vi "SICMDisplayGraph.vi"(6 "Baseline":dbl, 7 "Data":i16[](array[numeric]), 8 "TriggerHeight":dbl, 9 "TimeRes":cluster{"feedbackHz":u32, "memorywWriteDec":u16}, 10 "voltageRange":dbl, 11 "ArrayToReplace":waveform(dbl)[](array[waveform])) -> (3 "Graph":waveform(dbl)[](array[waveform]))   [LabVIEW 2016]
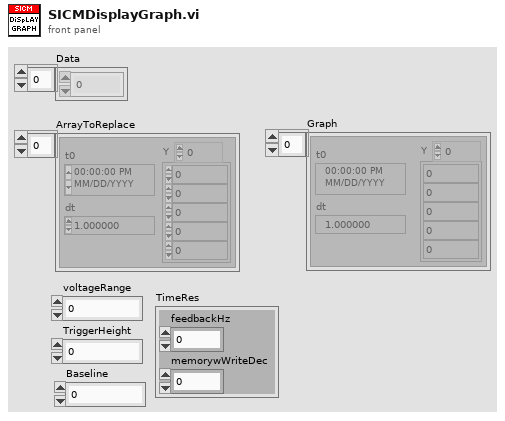
[diagram p1: front panel]
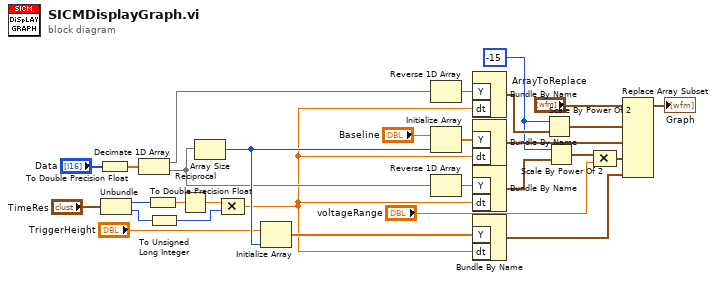
[diagram p0: block diagram]
diagram:
  w8 = i16 -15 ("n")
  n1 = To Double Precision Float(number="Data") -> (double precision float=w21:dbl[])
  n2 = Unbundle("TimeRes") -> ("feedbackHz"=w4:u32, "memorywWriteDec"=w2:u16)
  n3 = Decimate 1D Array(w21) -> (w11:dbl[], w13:dbl[])
  n4 = To Double Precision Float(number=w4) -> (double precision float=w7:dbl)
  n5 = To Unsigned Long Integer(number=w2) -> (unsigned 32bit integer=w1:u32)
  n6 = Reciprocal(x=w7) -> (1/x=w6:dbl)
  n7 = Array Size(array=w13) -> (size(s)=w15:i32)
  n8 = Compound Arithmetic op=MULTIPLY(w6, w1) -> (w3:dbl)
  n9 = Initialize Array("TriggerHeight", w15) -> (w18:dbl[])
  n10 = Reverse 1D Array(array=w11) -> (reversed array=w23:dbl[])
  n11 = Initialize Array("Baseline", w15) -> (w12:dbl[])
  n12 = Reverse 1D Array(array=w13) -> (reversed array=w24:dbl[])
  n13 = Bundle By Name("Y"=w23, "dt"=w3) -> (w19:waveform(dbl))  [unwired: 1 in]
  n14 = Bundle By Name("Y"=w12, "dt"=w3) -> (w27:waveform(dbl))  [unwired: 1 in]
  n15 = Bundle By Name("Y"=w24, "dt"=w3) -> (w20:waveform(dbl))  [unwired: 1 in]
  n16 = Bundle By Name("Y"=w18, "dt"=w3) -> (w26:waveform(dbl))  [unwired: 1 in]
  n17 = Scale By Power Of 2(n=w8, x=w19) -> (x*2^n=w28:waveform(dbl))
  n18 = Scale By Power Of 2(n=w8, x=w20) -> (x*2^n=w17:waveform(dbl))
  n19 = Compound Arithmetic op=MULTIPLY(w17, "voltageRange") -> (w25:waveform(dbl))
  n20 = Replace Array Subset(array="ArrayToReplace", new element #1=w28, new element #2=w27, new element #3=w25, new element #4=w26) -> (→"Graph":waveform(dbl)[])  [unwired: 4 in]
